vi "MQTT_Connect.vi"(4 "timeout ms (20000)":i32=20000, 5 "Connect Meta":T5={"QoS"=enum."At most once", "DUP"=FALSE, "Retain"=TRUE, "Keep Alive (sec)"=60}, 6 "Client ID":string="NodeE-12345", 7 "Connect Flags":T8={"user name"=FALSE, "password"=FALSE, "will retain"=TRUE, "will flag"=FALSE, "clean session"=FALSE, "reserved"=FALSE, "will QoS"=enum."At most once"}, 8 "error in (no error)":errorcluster, 9 "Will Info":T6={"Will message"="Last Will", "Will Topic"="Will Topic"}, 10 "User Info":T7={"User Name"="User", "Password"="password"}, 11 "MQTT Broker":cluster{"address (IP)":string, "port":u16}={"address (IP)"="broker.mqttdashboard.com", "port"=1883}) -> (0 "error out":errorcluster, 2 "Connection Status":T1=enum."Connection refused: not authorized", 3 "connection ID out":refnum<k5>)   [LabVIEW 2018, in "MQTT_Functions.lvlib"]
uses:
  MQTT_Functions.lvlib
  Controls/Connect_Flags.ctl
  Controls/QoS.ctl
  Controls/User_Info.ctl
  Controls/Will_Info.ctl
  Controls/DUP_Flag.ctl
  Controls/Retain_Flag.ctl
  Controls/Connection_Return_Codes.ctl
  Controls/MessageType.ctl
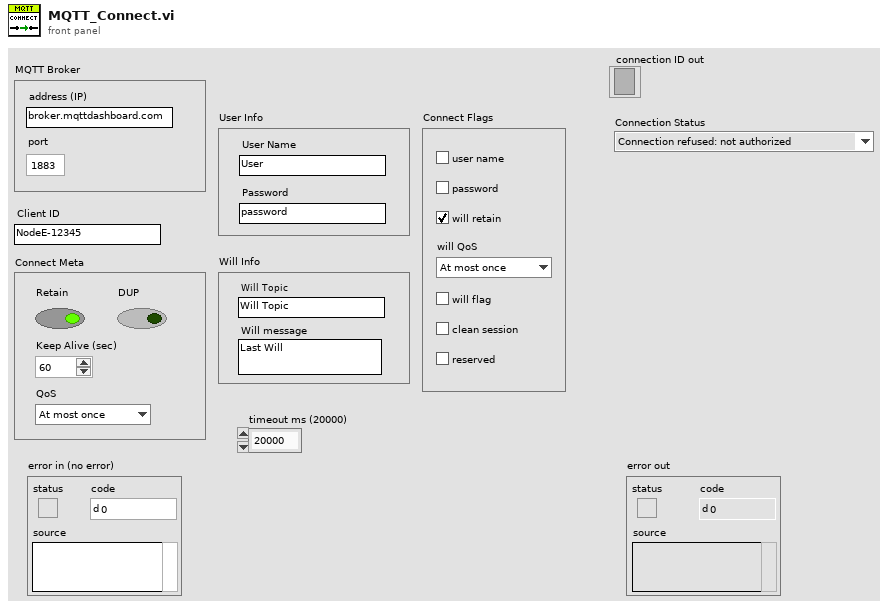
[diagram p1: front panel]
types:
  T1 = typedef "MQTT_Functions.lvlib/Connection_Return_Codes.ctl" = enum16{"Connection accepted", "Connection refused: unacceptable protocol version", "Connection refused: identifier rejected", "Connection refused: Server unavailable", "Connection refused: bad user name or password", "Connection refused: not authorized"}
  T2 = typedef "MQTT_Functions.lvlib/QoS.ctl" = enum8{"At most once", "At least once", "Exactly once", "Reserved"}
  T3 = typedef "MQTT_Functions.lvlib/DUP_Flag.ctl" = bool
  T4 = typedef "MQTT_Functions.lvlib/Retain_Flag.ctl" = bool
  T5 = cluster{"QoS":T2, "DUP":T3, "Retain":T4, "Keep Alive (sec)":u16}
  T6 = typedef "MQTT_Functions.lvlib/Will_Info.ctl" = cluster{"Will message":string, "Will Topic":string}
  T7 = typedef "MQTT_Functions.lvlib/User_Info.ctl" = cluster{"User Name":string, "Password":string}
  T8 = typedef "MQTT_Functions.lvlib/Connect_Flags.ctl" = cluster{"user name":bool, "password":bool, "will retain":bool, "will flag":bool, "clean session":bool, "reserved":bool, "will QoS":T2}
  T9 = typedef "MQTT_Functions.lvlib/MessageType.ctl" = enum32{"Reserved", "CONNECT", "CONNACK", "PUBLISH", "PUBACK", "PUBREC", "PUBREL", "PUBCOMP", "SUBSCRIBE", "SUBACK", "UNSUBSCRIBE", "UNSUBACK", "PINGREQ", "PINGRESP", "DISCONNECT", "Reserved2"}
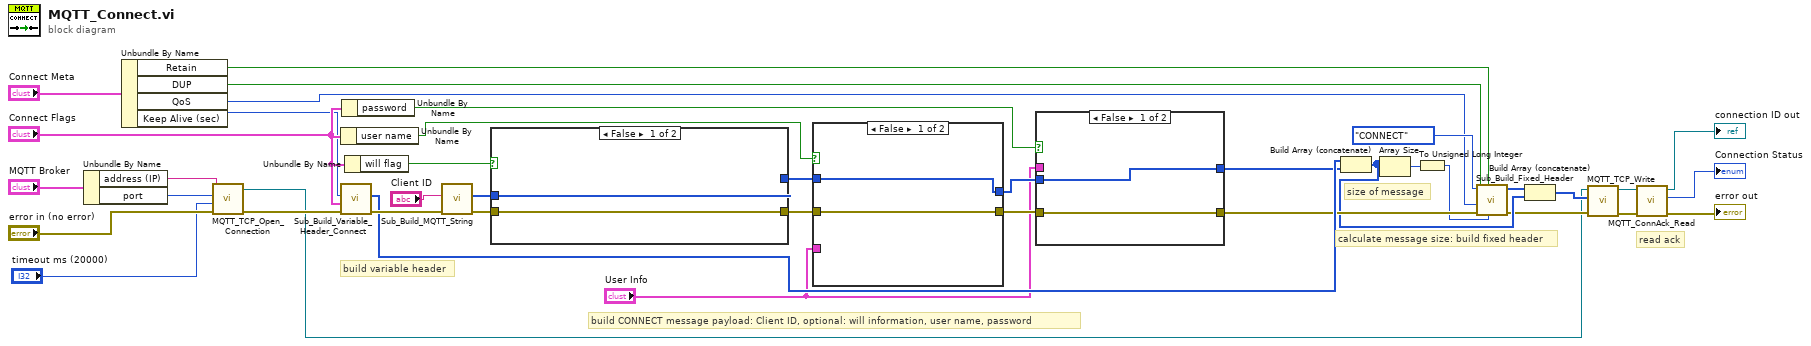
[diagram p0: block diagram]
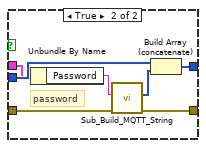
[diagram p2: hidden frame]
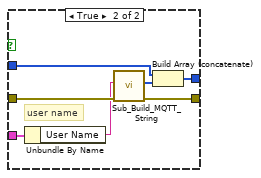
[diagram p3: hidden frame]
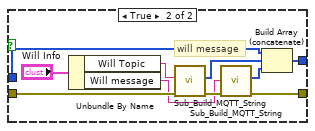
[diagram p4: hidden frame]
diagram:
  # "read ack"
  # "calculate message size: build fixed header"
  # "build CONNECT message payload: Client ID, optional: will information, user name, password"
  # "build variable header"
  # "size of message"
  n1 = Unbundle By Name("MQTT Broker") -> ("address (IP)"=w8:string, "port"=w2:u16)
  n2 = Unbundle By Name("Connect Meta") -> ("Retain"=w19:T4, "DUP"=w18:T3, "QoS"=w17:T2, "Keep Alive (sec)"=w16:u16)
  n3 = call "MQTT_TCP_Open_Connection.vi"("error in (no error)"="error in (no error)", "timeout ms (20000)"="timeout ms (20000)", "remote port or service name"=w2, "address"=w8) -> ("error out"=w11:errorcluster, "connection ID"=w10:refnum<k5>)  [unwired: 6 in]
  n4 = Unbundle By Name("Connect Flags") -> ("user name"=w33:bool)
  n5 = call "Sub_Build_Variable_Header_Connect.vi"("error in (no error)"=w11, "Connect Flags"="Connect Flags", "Keep Alive (sec)"=w16) -> ("error out"=w39:errorcluster, "Variable Header"=w30:u8[])  [unwired: 7 in]
  n6 = Unbundle By Name("Connect Flags") -> ("password"=w32:bool)
  n7 = Unbundle By Name("Connect Flags") -> ("will flag"=w31:bool)
  n8 = call "Sub_Build_MQTT_String.vi"("error in (no error)"=w39, "String to be encoded"="Client ID") -> ("error out"=w35:errorcluster, "UTF8 Byte Array"=w38:u8[])  [unwired: 8 in]
  n9 = case shown="False" w31 {
    tunnel: w38 -> [w42 w50]
    tunnel: [w42 w51] -> w37
    tunnel: w35 -> [w41 w49]
    tunnel: [w41 w46] -> w28
    frame False {
    }
    frame True {
      # "will message"
      n10 = Unbundle By Name("Will Info") -> ("Will Topic"=w44:string, "Will message"=w43:string)
      n11 = call "Sub_Build_MQTT_String.vi"("error in (no error)"=w49, "String to be encoded"=w44) -> ("error out"=w48:errorcluster, "UTF8 Byte Array"=w47:u8[])  [unwired: 8 in]
      n12 = call "Sub_Build_MQTT_String.vi"("error in (no error)"=w48, "String to be encoded"=w43) -> ("error out"=w46:errorcluster, "UTF8 Byte Array"=w52:u8[])  [unwired: 8 in]
      n13 = Build Array (concatenate)(w50, w47, w52) -> (w51:u8[])
    }
  }
  n14 = case shown="False" w33 {
    tunnel: w37 -> [w54 w60]
    tunnel: [w54 w59] -> w36
    tunnel: [w53 w58] -> w29
    tunnel: w28 -> [w53 w57]
    tunnel: "User Info" -> [_ w56]
    frame False {
    }
    frame True {
      # "user name"
      n15 = Unbundle By Name(w56) -> ("User Name"=w55:string)
      n16 = call "Sub_Build_MQTT_String.vi"("error in (no error)"=w57, "String to be encoded"=w55) -> ("error out"=w58:errorcluster, "UTF8 Byte Array"=w61:u8[])  [unwired: 8 in]
      n17 = Build Array (concatenate)(w60, w61) -> (w59:u8[])
    }
  }
  n18 = case shown="False" w32 {
    tunnel: w36 -> [w63 w69]
    tunnel: [w63 w68] -> w26
    tunnel: w29 -> [w62 w67]
    tunnel: [w62 w66] -> w27
    tunnel: "User Info" -> [_ w65]
    frame False {
    }
    frame True {
      # "password"
      n19 = Unbundle By Name(w65) -> ("Password"=w64:string)
      n20 = call "Sub_Build_MQTT_String.vi"("error in (no error)"=w67, "String to be encoded"=w64) -> ("error out"=w66:errorcluster, "UTF8 Byte Array"=w70:u8[])  [unwired: 8 in]
      n21 = Build Array (concatenate)(w69, w70) -> (w68:u8[])
    }
  }
  n22 = Build Array (concatenate)(w30, w26) -> (w25:u8[])
  n23 = Array Size(array=w25) -> (size(s)=w23:i32)
  n24 = To Unsigned Long Integer(number=w23) -> (unsigned 32bit integer=w22:u32)
  n25 = call "Sub_Build_Fixed_Header.vi"("Remaining Length"=w22, "Retain"=w19, "error in (no error)"=w27, "QoS"=w17, "DUP"=w18, "MessageType"=MessageType."CONNECT") -> ("error out"=w14:errorcluster, "Fixed Header"=w24:u8[])  [unwired: 4 in]
  n26 = Build Array (concatenate)(w24, w25) -> (w13:u8[])
  n27 = call "MQTT_TCP_Write.vi"("error in (no error)"=w14, "data in"=w13, "connection ID"=w10) -> ("error out"=w7:errorcluster, "connection ID out"=w6:refnum<k5>)  [unwired: 6 in, 1 out]
  n28 = call "MQTT_ConnAck_Read.vi"("error in (no error)"=w7, "connection ID"=w6) -> ("error out"=→"error out":errorcluster, "Connection Status"=→"Connection Status":T1, "connection ID out"=→"connection ID out":refnum<k5>)  [unwired: 5 in, 2 out]
